vi "Write OnOff Status (Single).vi"(8 "error in":errorcluster, 9 "Channel Index":i32, 10 "OnOff":bool, 11 "Cycler in":refnum<class "Cycler.lvclass">) -> (0 "error out":errorcluster, 3 "Cycler out":refnum<class "Cycler.lvclass">)   [LabVIEW 2023, in "Cycler.lvclass"]
uses:
  Cycler.lvclass
  Cycler.lvclass/Cycler.ctl
  <vilib>/ADAS Replay HIL/Channels/Tag Wrapper/Tag Wrapper.lvlib
  <vilib>/ADAS Replay HIL/Channels/Tag Wrapper/Polymorphic/Write Channel (Boolean).vi
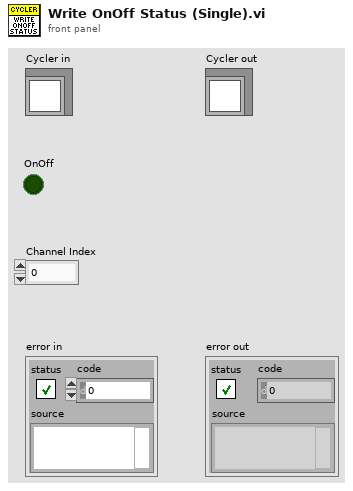
[diagram p1: front panel]
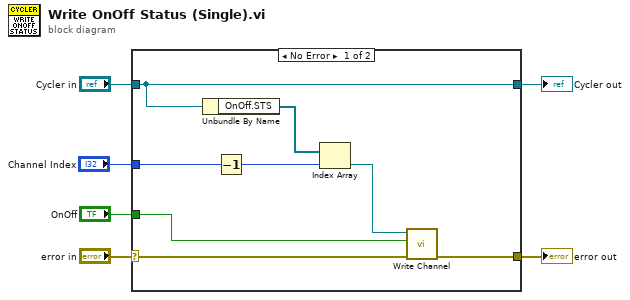
[diagram p0: block diagram]
diagram:
  n1 = case shown="No Error" "error in" {
    selector: "error in" -> [w13 w15]
    tunnel: [w12 w15] -> w5
    tunnel: [w14 w16] -> w3
    tunnel: "Cycler in" -> [w14 w16]
    tunnel: "OnOff" -> [w10 _]
    tunnel: "Channel Index" -> [w8 _]
    frame No Error {
      n2 = Unbundle By Name(w14) -> ("OnOff.STS"=w11:refnum<k21>[])
      n3 = Decrement(x=w8) -> (x-1=w7:i32)
      n4 = Index Array(array=w11, index=w7) -> (element=w9:refnum<k21>)
      n5 = call-poly <vilib>:"Write Channel.vi"("error in"=w13, "Value to Write"=w10, "ADAS HIL Channel in"=w9) -> ("error out"=w12:errorcluster)  [unwired: 6 in, 2 out]
    }
    frame Error {
    }
  }
  "error out" <- w5
  "Cycler out" <- w3
